vi "Log Tool Config Rtn Event Helper.vi"(7 "State Info":string, 8 "error in (no error)":errorcluster, 9 "Tool Type":i32, 10 "Connecting":bool, 11 "EventLog in":refnum<class "EventLog.lvclass">) -> (0 "error out":errorcluster, 3 "EventLog out":refnum<class "EventLog.lvclass">)   [LabVIEW 2015, in "Tool Module.lvlib"]
uses:
  Tool Module.lvlib
  QC-X App/Libraries/Event Logger Library/Event Log/EventLog.lvclass
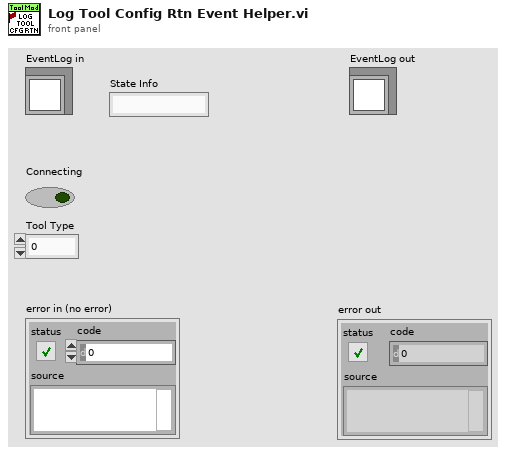
[diagram p1: front panel]
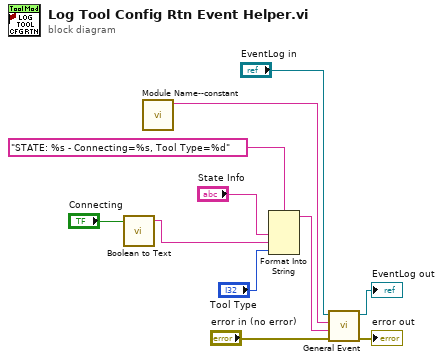
[diagram p0: block diagram]
diagram:
  n1 = call "Boolean to Text.vi"("selector"="Connecting") -> ("output string"=w11:string)  [unwired: 4 in]
  n2 = call "Module Name--constant.vi"() -> ("Module Name"=w1:string)  [unwired: 11 in]
  n3 = Format Into String(format string="STATE: %s - Connecting=%s, Tool Type=%d", "State Info", w11, "Tool Type") -> (resulting string=w9:string)  [unwired: 2 in, 1 out]
  n4 = call "General Event.vi"("error in (no error)"="error in (no error)", "Event Description"=w9, "Event Name"=w1, "EventLog ref"="EventLog in") -> ("error out"=→"error out":errorcluster, "EventLog ref"=→"EventLog out":refnum<class "EventLog.lvclass">)  [unwired: 6 in]
